vi "uarttest.vi"() -> ()   [LabVIEW 2019]
uses:
  <vilib>/myRIO/Instrument Drivers/Onboard IO/UART/typedef/VISA Configuration.ctl
  KNRm_ReMi_OS6.lvlibp/KNRm_ReMi_Toolkit/IO/LowLevel/IO_Channel_DIO.ctl
  KNRm_ReMi_OS6.lvlibp/KNRm_ReMi_Toolkit/Control/MotorNumberSelect.ctl
  <vilib>/Instr/_visa.llb/VISA Configure Serial Port (Instr).vi
  <vilib>/myRIO/Express VI/Onboard IO/UART/UART Express VI.xnode
  <vilib>/myRIO/Instrument Drivers/Onboard IO/UART/UART.lvlib
  KNRm_ReMi_OS6.lvlibp
  <vilib>/Platform/TimedLoop/XDataNode/XDataNode.xnode
  <vilib>/Platform/TimedLoop/XDataNode/nitl_modes.ctl
  <vilib>/Platform/TimedLoop/XDataNode/XDNodeRunTimeDep.lvlib
  <vilib>/Platform/TimedLoop/XDataNode/wakeup.ctl
  <vilib>/Platform/TimedLoop/XDataNode/timing_clust.ctl
  SJCube_Lib/SJCube Folder/SJCube.lvlib
  <vilib>/addons/control/pid/NI_PID_pid.lvlib
  <vilib>/addons/control/pid/pid.llb/PID (DBL).vi
panel:
  out "Array":string[](array[string])
  out "output":dbl format="%.2f"
  out "Numeric Control":i32
  out "x-y":dbl
  in  "Stop Button 3":bool
  out "Position(deg)":dbl(knob) scale=80.0..-80.0
  in  "Reset":bool
  in  "Stop Button 2":bool
  in  "PosPID":T1={"proportional gain (Kc)"=-0.05999999999999999, "integral time (Ti, min)"=0.03, "derivative time (Td, min)"=0.019999999999999997}
  out "Waveform Chart":T2(graph)
  in  "Setpoint(deg)":dbl(knob) scale=80.0..-80.0
  in  "BalancePID":T1={"proportional gain (Kc)"=0.07999999999999999, "integral time (Ti, min)"=0.0, "derivative time (Td, min)"=0.0008}
  in  "Auto\nSetpoint":bool
  in  "x":bool
  in  "W":string[](array[string])
  out "R":string[](array[string])
  out "ENC(Deg)":dbl
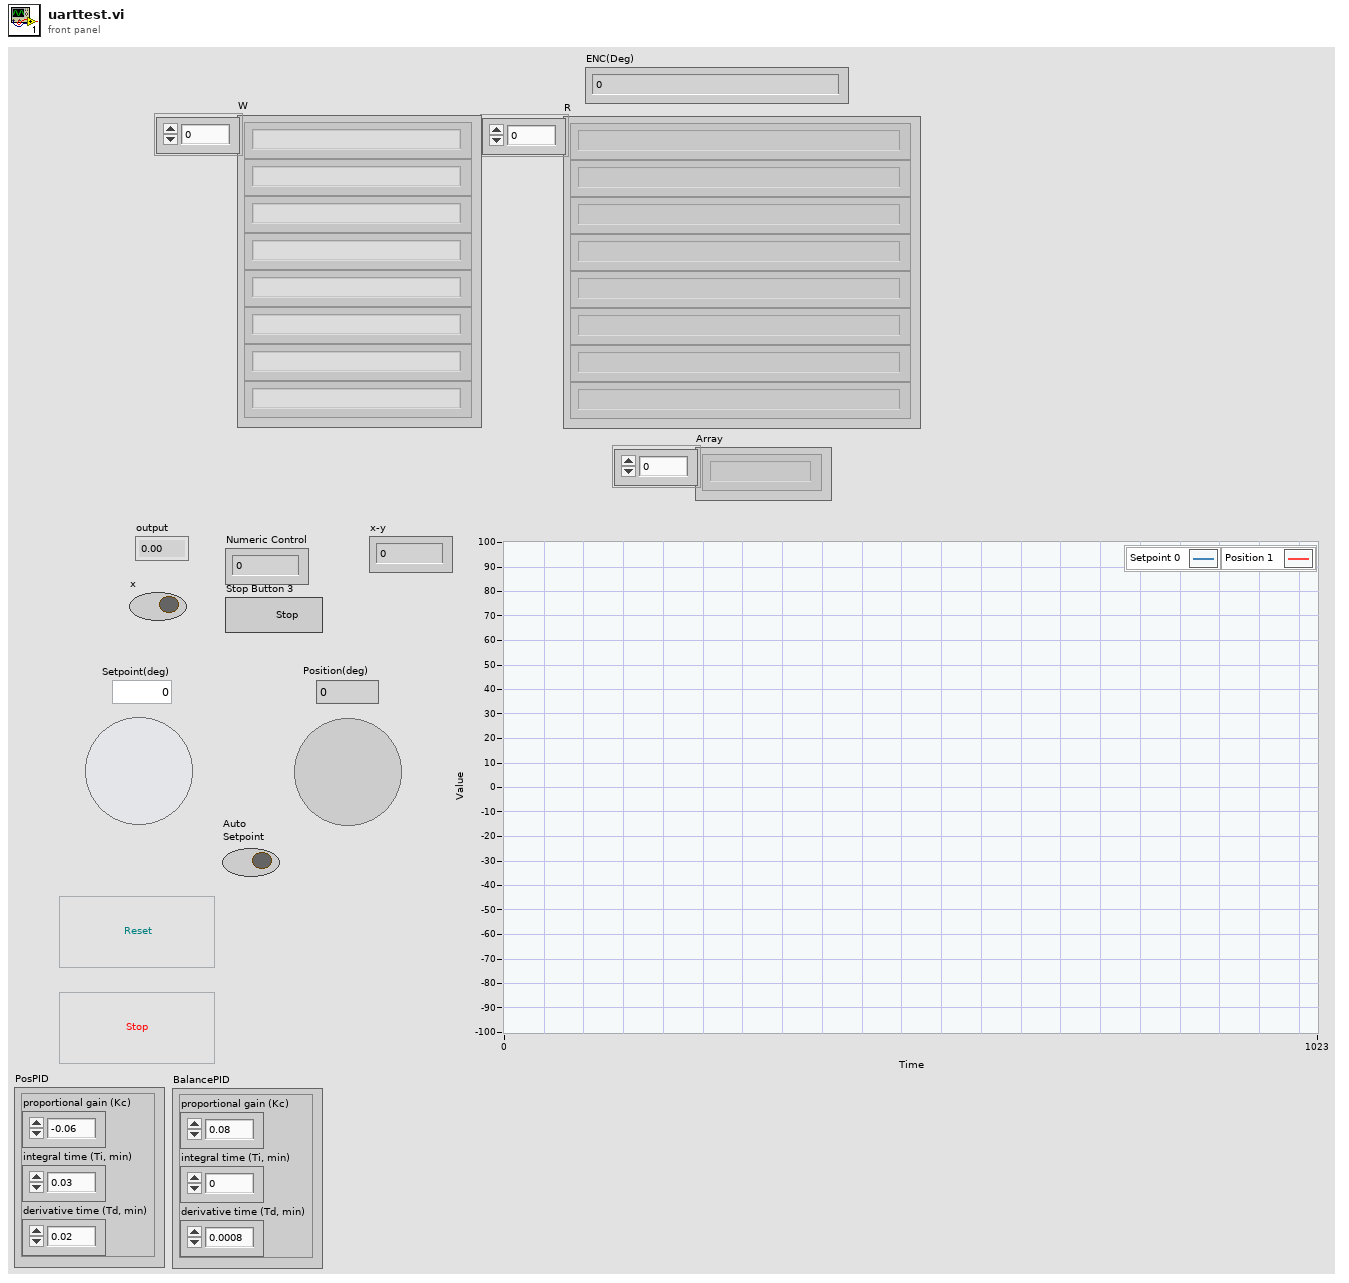
[diagram p1: front panel]
types:
  T1 = cluster{"proportional gain (Kc)":dbl, "integral time (Ti, min)":dbl, "derivative time (Td, min)":dbl}
  T2 = cluster{"Setpoint(deg)":dbl, "PresentPOS(deg)":dbl}
  T3 = typedef "UART.lvlib/VISA Configuration.ctl" = cluster{"baud rate (9600)":u32, "data bits (8)":u16, "parity (0:none)":enum16{"None", "Odd", "Even", "Mark", "Space"}, "stop bits (10: 1 bit)":u16, "flow control (0:none)":u16, "termination char\n(0xA = '\\n' = LF) ":u8, "Enable Termination\nChar (T)":bool, "timeout (10sec)":u32}
  T4 = typedef "KNRm_ReMi_OS6.lvlibp/MotorNumberSelect.ctl" = enum16{"DS1", "DS2", "DS3", "DS4"}
  T5 = typedef "KNRm_ReMi_OS6.lvlibp/IO_Channel_DIO.ctl" = enum16{"B/DIO1 (M1)", "A/DIO8 (M2)", "B/DIO7 (M3)", "A/DIO3 (M4)", "A/DIO14 (RC1_0)", "A/DIO15 (RC1_1)", "A/DIO7(S1)", "A/DIO2(S2)", "A/DIO6(S3)", "A/DIO3(S4)", "A/DIO5(S5)", "A/DIO4(S6)"}
  T6 = typedef "XDNodeRunTimeDep.lvlib/timing_clust.ctl" = cluster{"Expected End [f-1]":u64, "Actual End [f-1]":u64, "Finished Late? [f-1]":bool, "Expected End [i-1]":u64, "Actual End [i-1]":u64, "Finished Late? [i-1]":bool, "Expected Start [i]":u64, "Actual Start [i]":u64, "Expected Start [f]":u64, "Actual Start [f]":u64, "Source Name":string, "Structure Name":string, "Period":i64, "Deadline":i64, "Offset":i64, "Start":i64, "Priority":i32, "Timeout":i32, "Mode":T7, "Wakeup Reason":T8, "Error":errorcluster, "Source Type":string, "Secondary Source Type":string, "Global End Time":u64, "Global Start Time":u64, "Frame Duration":u64, "Iteration Duration":u64, "Assigned CPU":i32, "I/O Scan Engine Mode":u32}
  T7 = typedef "XDNodeRunTimeDep.lvlib/nitl_modes.ctl" = enum32{"No Change", "Process missed periods, maintain original phase", "Discard missed periods, maintain original phase", "Process missed periods, ignore original phase", "Discard missed periods, ignore original phase"}
  T8 = typedef "XDNodeRunTimeDep.lvlib/wakeup.ctl" = enum32{"Normal", "Aborted", "Asynchronous wakeup", "Timing source error", "Timed loop error", "Timeout"}
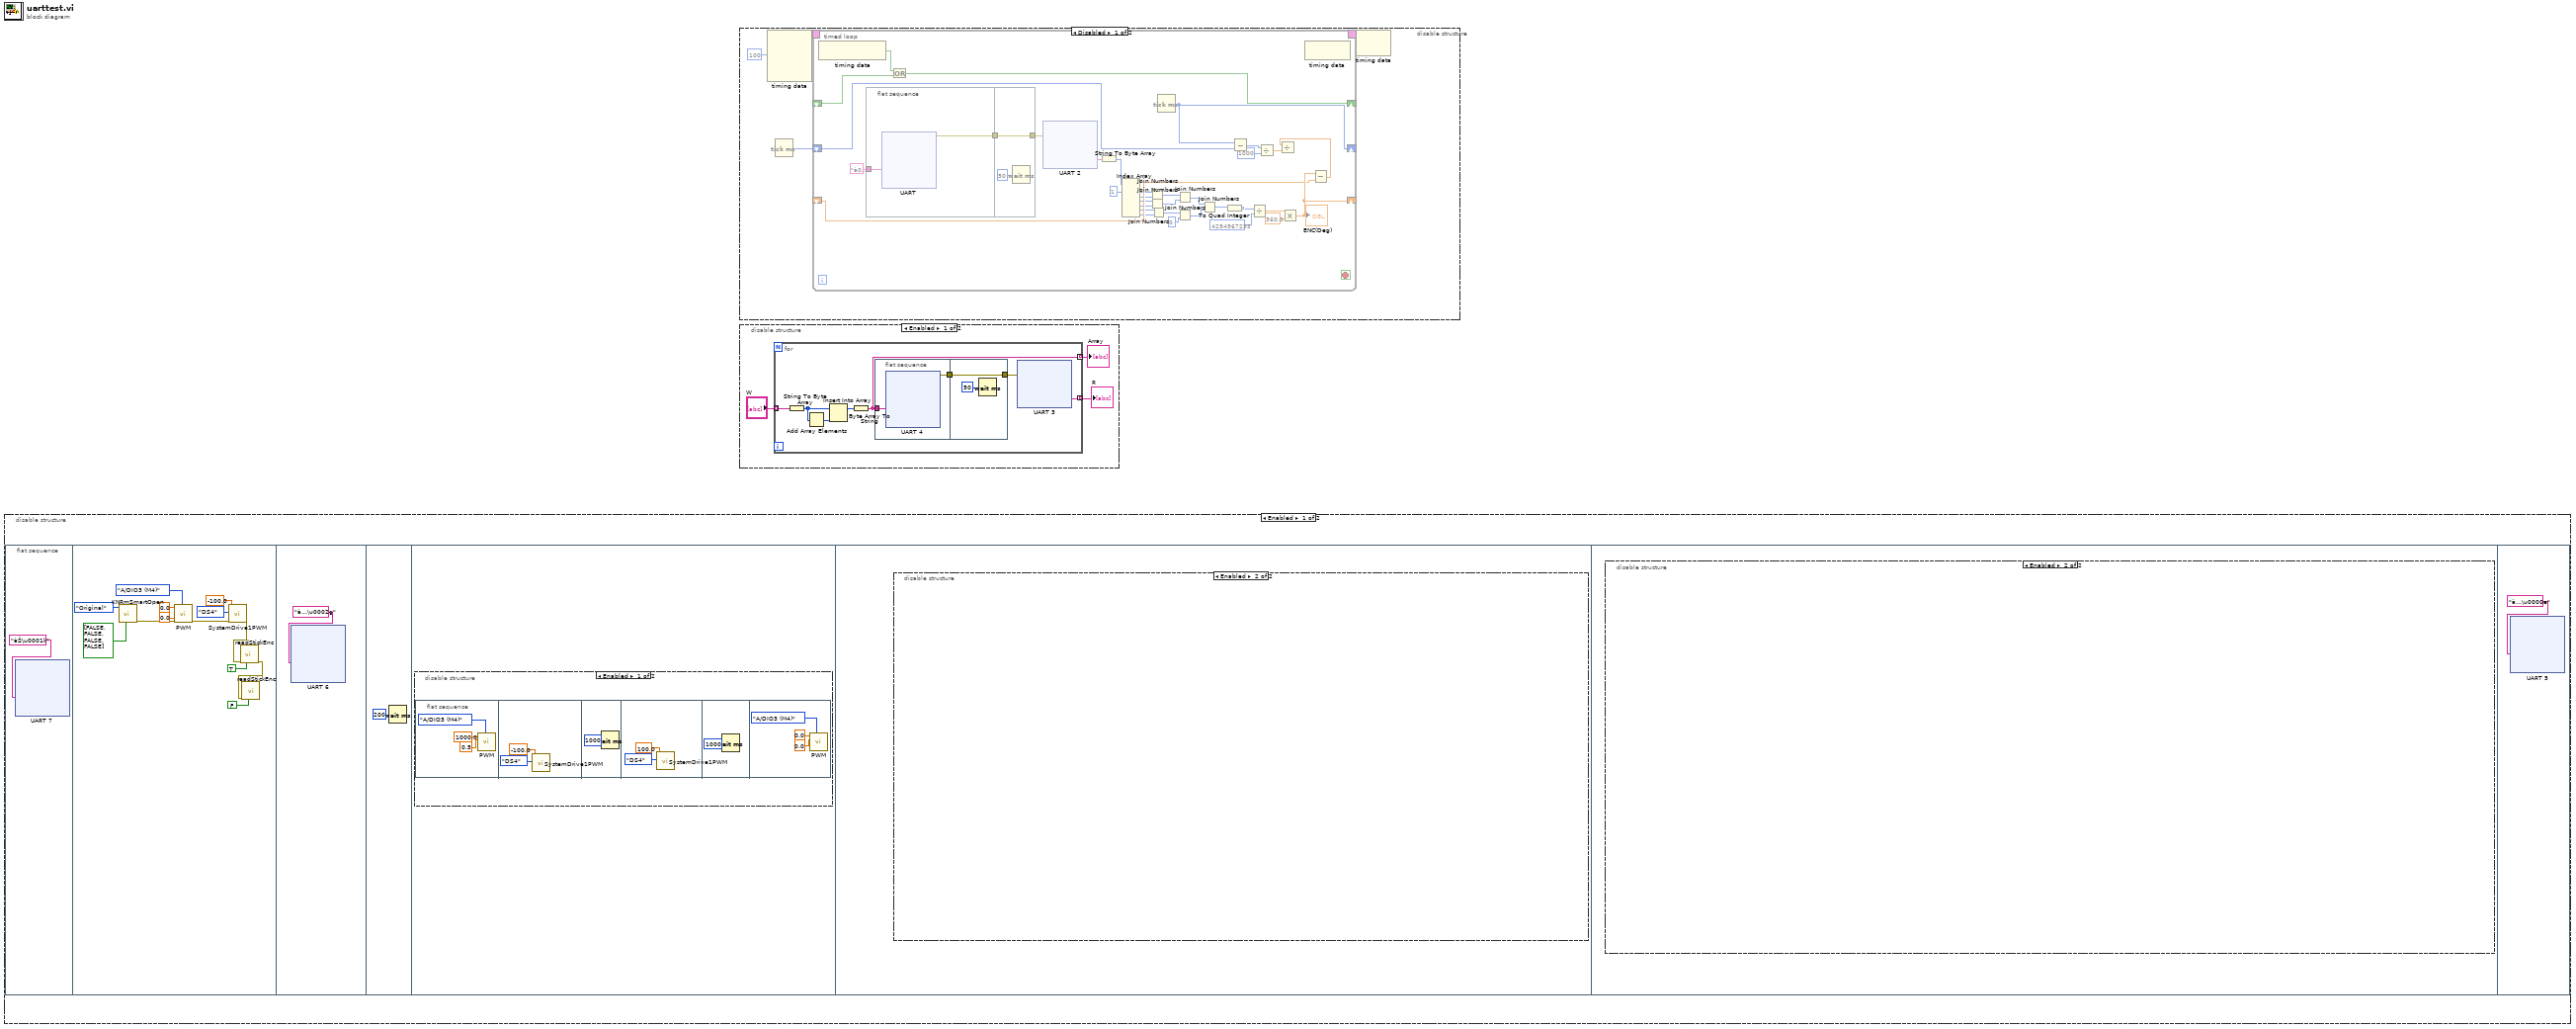
[diagram p0: block diagram]
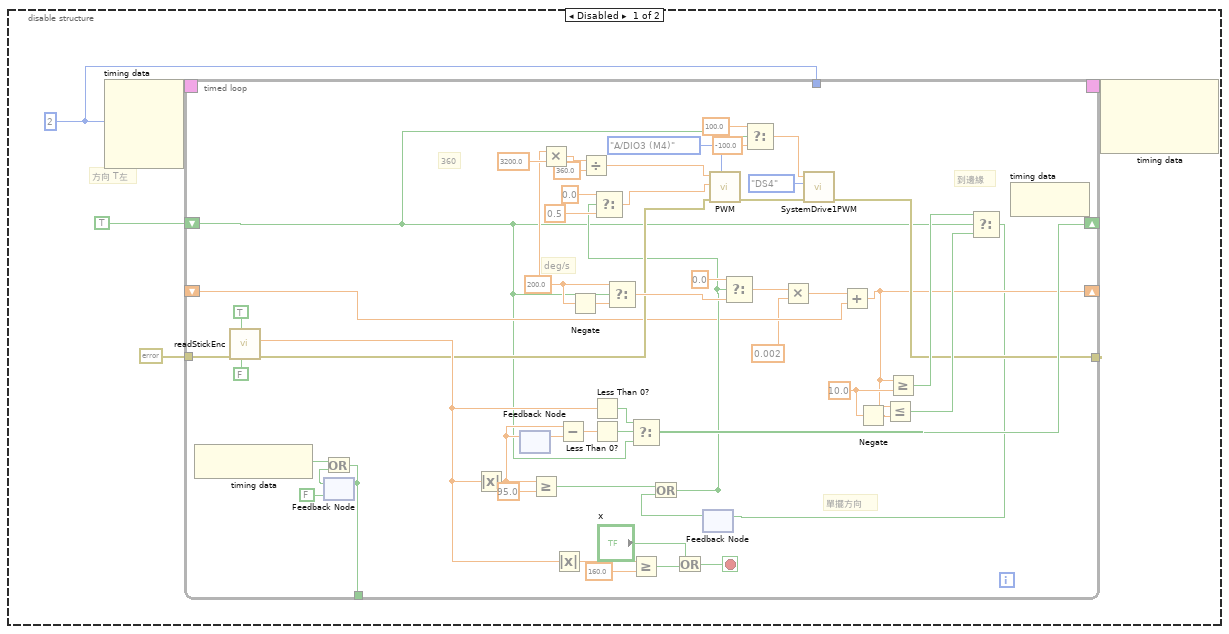
[diagram p3: hidden frame]
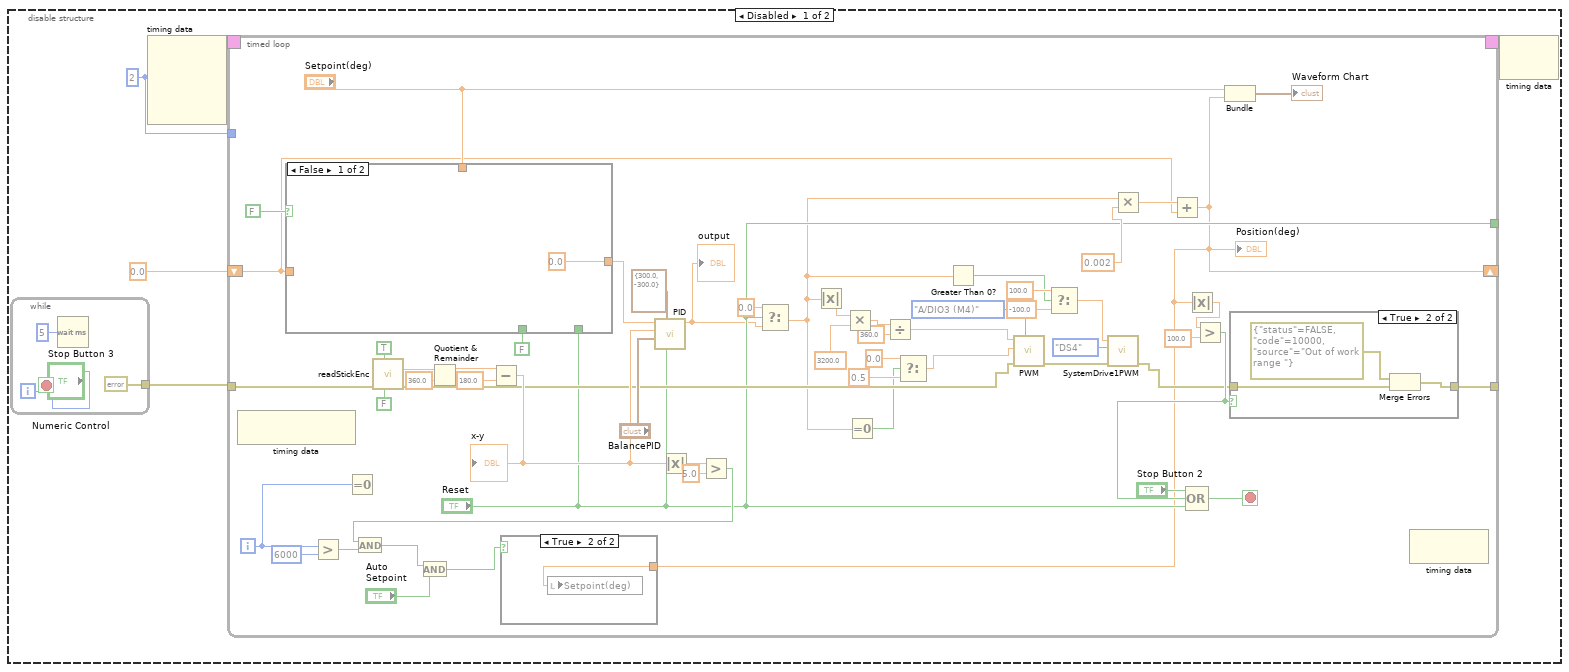
[diagram p4: hidden frame]
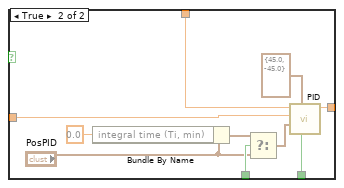
[diagram p6: hidden frame]
diagram:
  n1 = disable-structure shown="Enabled" {
    frame Enabled {
      n2 = flat-sequence {
        frame #0 {
          n3 = xnode "UART 7"("Characters to Write"="àŠ\u0001k" ("string")) -> ()  [unwired: 1 in, 2 out]
        }
        frame #1 {
          n4 = call "KNRmSmartOpen.vi"("SpeedMode"=bool[] [FALSE, FALSE, FALSE, FALSE], "INI FPGA MODE"=enum16{"Original", "M4EXTIOB"}."Original") -> ("error out"=w24:errorcluster)  [unwired: 6 in, 3 out]
          n5 = call "PWM.vi"("IO_Chanel"=IO_Channel_DIO."A/DIO3 (M4)", "error in"=w24, "DutyCycle"=0.0, "Frequency(Hz)"=0.0) -> ("error out"=w23:errorcluster)  [unwired: 7 in]
          n6 = call "SystemDrive1PWM.vi"("error in"=w23, "MotorNumberSelect"=MotorNumberSelect."DS4", "MotorSpeed(PWM%)"=-100.0) -> ("error out"=w29:errorcluster)  [unwired: 7 in, 1 out]
          n7 = call "readStickEnc.vi"("Reset Counter"=TRUE, "error in (no error)"=w29) -> ("error out"=w30:errorcluster)  [unwired: 8 in, 1 out]
          n8 = call "readStickEnc.vi"("Reset Counter"=FALSE, "error in (no error)"=w30) -> ()  [unwired: 8 in, 2 out]
        }
        frame #2 {
          n9 = xnode "UART 6"("Characters to Write"="à…\u0002g" ("string")) -> ()  [unwired: 1 in, 2 out]
        }
        frame #3 {
          n10 = Wait (ms)(milliseconds to wait=u32 200) -> ()  [unwired: 1 out]
        }
        frame #4 {
          n11 = disable-structure shown="Enabled" {
            frame Enabled {
              n12 = flat-sequence {
                frame #0 {
                  n13 = call "PWM.vi"("IO_Chanel"=IO_Channel_DIO."A/DIO3 (M4)", "DutyCycle"=0.5, "Frequency(Hz)"=1000.0) -> ()  [unwired: 8 in, 1 out]
                }
                frame #1 {
                  n14 = call "SystemDrive1PWM.vi"("MotorNumberSelect"=MotorNumberSelect."DS4", "MotorSpeed(PWM%)"=-100.0) -> ()  [unwired: 8 in, 2 out]
                }
                frame #2 {
                  n15 = Wait (ms)(milliseconds to wait=u32 1000) -> ()  [unwired: 1 out]
                }
                frame #3 {
                  n16 = call "SystemDrive1PWM.vi"("MotorNumberSelect"=MotorNumberSelect."DS4", "MotorSpeed(PWM%)"=100.0) -> ()  [unwired: 8 in, 2 out]
                }
                frame #4 {
                  n17 = Wait (ms)(milliseconds to wait=u32 1000) -> ()  [unwired: 1 out]
                }
                frame #5 {
                  n18 = call "PWM.vi"("IO_Chanel"=IO_Channel_DIO."A/DIO3 (M4)", "DutyCycle"=0.0, "Frequency(Hz)"=0.0) -> ()  [unwired: 8 in, 1 out]
                }
              }
            }
            frame Disabled {
            }
          }
        }
        frame #5 {
          n19 = disable-structure shown="Enabled" {
            frame Disabled {
              w61 = i64 2 ("Period")
              # "方向 T左"
              n20 = node-c288(w61) -> (w66:T6)  [unwired: 3 in]
              n21 = timed-loop {
                timing: w66 -> [_]
                timing-out: [_] -> w65
                tunnel: errorcluster {"status"=FALSE, "code"=0, "source"=""} ("error in (no error)") -> [w113]
                tunnel: [w86] -> _
                tunnel: w61 -> [_]
                shift-right: [w100] -> _
                shift-left: TRUE -> [w69]
                tunnel: [w96] -> w64
                shift-right: [w72] -> _
                shift-left: _ -> [w74]
                stop <- w117 stop-if-true
                w95 = 10.0 ("UpLimit")
                w78 = 200.0
                # "360"
                # "deg/s"
                # "單擺方向"
                # "到邊緣"
                n22 = node-c288() -> (w99:bool)  [unwired: 1 in]
                n23 = call "readStickEnc.vi"("Reset Counter"=FALSE, "Reverse ENC?"=TRUE, "error in (no error)"=w113) -> ("error out"=w87:errorcluster, "StickEncoder (deg)"=w93:dbl)  [unwired: 7 in]
                n24 = feedback #1(FALSE) -> (w98:bool)
                n25 = Or(x=w99, y=w98) -> (x .or. y?=w96:bool)
                n26 = feedback-in #1(w96) -> ()
                n27 = Absolute Value(x=w93) -> (abs(x)=w104:dbl)
                n28 = feedback-in #2(w104) -> ()
                n29 = feedback #2() -> (w108:dbl)  [unwired: 1 in]
                n30 = Greater Or Equal?(x=w104, y=95.0) -> (x >= y?=w106:bool)
                n31 = Multiply(x=w78, y=3200.0) -> (x*y=w82:dbl)
                n32 = Absolute Value(x=w93) -> (abs(x)=w119:dbl)
                n33 = Subtract(x=w104, y=w108) -> (x-y=w107:dbl)
                n34 = Negate(x=w78) -> (-x=w110:dbl)
                n35 = Divide(x=w82, y=360.0) -> (x/y=w79:dbl)
                n36 = Less Than 0?(x=w93) -> (x < 0?=w102:bool)
                n37 = Less Than 0?(x=w107) -> (x < 0?=w103:bool)
                n38 = Select(t=w78, s=w69, f=w110) -> (s? t:f=w91:dbl)
                n39 = Select(t=w102, s=w103, f=w69) -> (s? t:f=w100:bool)
                n40 = Greater Or Equal?(x=w119, y=160.0) -> (x >= y?=w101:bool)
                n41 = Or(x="x", y=w101) -> (x .or. y?=w117:bool)
                n42 = feedback #3() -> (w105:bool)  [unwired: 1 in]
                n43 = Or(x=w106, y=w105) -> (x .or. y?=w77:bool)
                n44 = Select(t=0.0, s=w77, f=0.5 ("DutyCycle")) -> (s? t:f=w84:dbl)
                n45 = call "PWM.vi"("IO_Chanel"=IO_Channel_DIO."A/DIO3 (M4)", "error in"=w87, "DutyCycle"=w84, "Frequency(Hz)"=w79) -> ("error out"=w90:errorcluster)  [unwired: 7 in]
                n46 = Select(t=0.0, s=w77, f=w91) -> (s? t:f=w76:dbl)
                n47 = Select(t=100.0, s=w69, f=-100.0) -> (s? t:f=w70:dbl)
                n48 = Multiply(x=w76, y=0.002) -> (x*y=w75:dbl)
                n49 = call "SystemDrive1PWM.vi"("error in"=w90, "MotorNumberSelect"=MotorNumberSelect."DS4", "MotorSpeed(PWM%)"=w70) -> ("error out"=w86:errorcluster)  [unwired: 7 in, 1 out]
                n50 = Add(x=w75, y=w74) -> (x+y=w72:dbl)
                n51 = Negate(x=w95) -> (-x=w94:dbl)
                n52 = Less Or Equal?(x=w72, y=w94) -> (x <= y?=w115:bool)
                n53 = Greater Or Equal?(x=w72, y=w95) -> (x >= y?=w116:bool)
                n54 = Select(t=w116, s=w69, f=w115) -> (s? t:f=w71:bool)
                n55 = feedback-in #3(w71) -> ()
                n56 = node-c288() -> ()  [unwired: 1 in, 1 out]
              }
              n57 = node-c288(w65) -> ()  [unwired: 3 out]
            }
            frame Enabled {
            }
          }
        }
        frame #6 {
          n58 = disable-structure shown="Enabled" {
            frame Disabled {
              w129 = i64 2 ("Period")
              n59 = while {
                tunnel: [errorcluster {"status"=FALSE, "code"=0, "source"=""} ("error out")] -> w127
                i -> [w133]
                stop <- "Stop Button 3" stop-if-true
                n60 = Wait (ms)(milliseconds to wait=u32 5) -> ()  [unwired: 1 out]
                "Numeric Control" <- w133
              }
              n61 = node-c288(w129) -> (w131:T6)  [unwired: 3 in]
              n62 = timed-loop "Timed Loop" {
                timing: w131 -> [_]
                timing-out: [_] -> w130
                shift-right: [w140] -> _
                shift-left: 0.0 -> [w162]
                tunnel: w127 -> [w182]
                tunnel: ["Reset"] -> _
                tunnel: [w180] -> _
                tunnel: w129 -> [_]
                i -> [w166]
                stop <- w186 stop-if-true
                n63 = node-c288() -> ()  [unwired: 1 in, 1 out]
                n64 = case shown="False" FALSE ("StickPosControl") {
                  tunnel: [0.0 ("output") w202] -> w173
                  tunnel: w162 -> [_ w201]
                  tunnel: "Reset" -> [_ w200]
                  tunnel: "Setpoint(deg)" -> [_ w199]
                  tunnel: FALSE -> [_ w198]
                  frame False {
                  }
                  frame True {
                    n65 = Bundle By Name(cluster="PosPID", "integral time (Ti, min)"=0.0) -> (w195:T1)
                    n66 = Select(t=w195, s=w198, f="PosPID") -> (s? t:f=w197:T1)
                    n67 = call-poly <vilib>:"PID.vi"("reinitialize? (F)"=w200, "output range"=cluster{"output high":dbl, "output low":dbl} {"output high"=45.0, "output low"=-45.0}, "PID gains"=w197, "process variable"=w201, "setpoint"=w199) -> ("output"=w202:dbl)  [unwired: 5 in, 1 out]
                  }
                }
                n68 = Greater?(x=w166, y=6000) -> (0:w174:bool)
                n69 = Equal To 0?(x=w166) -> ()  [unwired: 1 out]
                n70 = call "readStickEnc.vi"("Reset Counter"=FALSE, "Reverse ENC?"=TRUE, "error in (no error)"=w182) -> ("error out"=w144:errorcluster, "StickEncoder (deg)"=w184:dbl)  [unwired: 7 in]
                n71 = Quotient & Remainder(x=w184, y=360.0) -> (x-y*floor(x/y)=w187:dbl)  [unwired: 1 out]
                n72 = Subtract(x=w187, y=180.0) -> (x-y=w170:dbl)
                "x-y" <- w170
                n73 = call-poly <vilib>:"PID.vi"("reinitialize? (F)"="Reset", "output range"=cluster{"output high":dbl, "output low":dbl} {"output high"=300.0, "output low"=-300.0}, "PID gains"="BalancePID", "process variable"=w170, "setpoint"=w173) -> ("output"=w136:dbl)  [unwired: 5 in, 1 out]
                "output" <- w136
                n74 = Absolute Value(x=w170) -> (abs(x)=w172:dbl)
                n75 = Greater?(x=w172, y=5.0) -> (0:w165:bool)
                n76 = And(x=w165, y=w174) -> (x .and. y?=w169:bool)
                n77 = And(x=w169, y="Auto\nSetpoint") -> (x .and. y?=w167:bool)
                n78 = Select(t=0.0, s="Reset", f=w136) -> (s? t:f=w138:dbl)
                n79 = Absolute Value(x=w138) -> (abs(x)=w137:dbl)
                n80 = Multiply(x=w137, y=3200.0) -> (x*y=w151:dbl)
                n81 = Equal To 0?(x=w138) -> (x = 0?=w139:bool)
                n82 = Divide(x=w151, y=360.0) -> (x/y=w148:dbl)
                n83 = Select(t=0.0, s=w139, f=0.5 ("DutyCycle")) -> (s? t:f=w153:dbl)
                n84 = Greater Than 0?(x=w138) -> (x > 0?=w142:bool)
                n85 = call "PWM.vi"("IO_Chanel"=IO_Channel_DIO."A/DIO3 (M4)", "error in"=w144, "DutyCycle"=w153, "Frequency(Hz)"=w148) -> ("error out"=w157:errorcluster)  [unwired: 7 in]
                n86 = Select(t=100.0, s=w142, f=-100.0) -> (s? t:f=w147:dbl)
                n87 = call "SystemDrive1PWM.vi"("error in"=w157, "MotorNumberSelect"=MotorNumberSelect."DS4", "MotorSpeed(PWM%)"=w147) -> ("error out"=w143:errorcluster)  [unwired: 7 in, 1 out]
                n88 = Multiply(x=w138, y=0.002) -> (x*y=w163:dbl)
                n89 = Add(x=w163, y=w162) -> (x+y=w140:dbl)
                "Position(deg)" <- w140
                n90 = case shown="True" w167 {
                  tunnel: w140 -> [_ w192]
                  frame False {
                  }
                  frame True {
                    n91 = local write "Setpoint(deg)"(w192) -> ()
                  }
                }
                n92 = Absolute Value(x=w140) -> (abs(x)=w160:dbl)
                n93 = Greater?(x=w160, y=100.0 ("WorkRange")) -> (0:w158:bool)
                n94 = Compound Arithmetic op=OR("Stop Button 2", w158, "Reset") -> (w186:bool)
                n95 = Bundle("Setpoint(deg)"="Setpoint(deg)", w140) -> (→"Waveform Chart":cluster{"Setpoint(deg)":dbl, dbl})  [unwired: 1 in]
                n96 = case shown="True" w158 {
                  tunnel: w143 -> [w204 w207]
                  tunnel: [w204 w205] -> w180
                  frame False {
                  }
                  frame True {
                    n97 = Merge Errors(errorcluster {"status"=FALSE, "code"=10000, "source"="Out of work range "} ("error in (no error)"), w207) -> (w205:errorcluster)
                  }
                }
                n98 = node-c288() -> ()  [unwired: 1 in, 1 out]
              }
              n99 = node-c288(w130) -> ()  [unwired: 1 out]
            }
            frame Enabled {
            }
          }
        }
        frame #7 {
          n100 = xnode "UART 5"("Characters to Write"="à…\u0000e" ("string")) -> ()  [unwired: 1 in, 2 out]
        }
      }
    }
    frame Disabled {
    }
  }
  n101 = disable-structure shown="Disabled" {
    frame Disabled {
      n102 = node-c288(i64 100 ("Period")) -> (w234:T6)  [unwired: 3 in]
      n103 = Tick Count (ms)() -> (millisecond timer value=w232:u32)
      n104 = timed-loop {
        shift-right: [w267] -> _
        shift-left: w232 -> [w268]
        shift-right: [w266] -> _
        shift-left: _ -> [w265]
        timing: w234 -> [_]
        timing-out: [_] -> w233
        shift-right: [w236] -> _
        shift-left: _ -> [w235]
        stop <- _ stop-if-true
        n105 = node-c288() -> (w237:bool)  [unwired: 1 in]
        n106 = flat-sequence {
          tunnel: "à0\u0010" ("string") -> [w270]
          tunnel: [w269] -> w264
          tunnel: [w288] -> w263
          tunnel: w264 -> [w288]
          frame #0 {
            n107 = xnode "UART"("Characters to Write"=w270) -> ("error out"=w269:errorcluster)  [unwired: 1 in, 1 out]
          }
          frame #1 {
            n108 = Wait (ms)(milliseconds to wait=u32 50) -> ()  [unwired: 1 out]
          }
        }
        n109 = Or(x=w237, y=w235) -> (x .or. y?=w236:bool)
        n110 = xnode "UART 2"("error in (no error)"=w263) -> ("Characters Read"=w262:string)  [unwired: 1 out]
        n111 = String To Byte Array(string=w262) -> (unsigned byte array=w261:u8[])
        n112 = Index Array(array=w261, index #1=1 ("index")) -> (element #1=w257:u8, element #2=w256:u8, element #3=w255:u8, element #4=w254:u8, element #5=w253:u8, element #6=w252:u8)  [unwired: 5 in]
        n113 = Join Numbers(hi=w257, lo=w256) -> ((hi.lo)=w251:u16)
        n114 = Join Numbers(hi=w255, lo=w254) -> ((hi.lo)=w250:u16)
        n115 = Join Numbers(hi=w253, lo=w252) -> ((hi.lo)=w249:u16)
        n116 = Tick Count (ms)() -> (millisecond timer value=w267:u32)
        n117 = Join Numbers(hi=w251, lo=w250) -> ((hi.lo)=w259:u32)
        n118 = Join Numbers(hi=w249, lo=u16 0) -> ((hi.lo)=w258:u32)
        n119 = Join Numbers(hi=w259, lo=w258) -> ((hi.lo)=w247:u64)
        n120 = To Quad Integer(1:w247) -> (0:w243:i64)
        n121 = Subtract(x=w267, y=w268) -> (x-y=w241:u32)
        n122 = Divide(x=w243, y=i64 4294967295) -> (x/y=w245:dbl)
        n123 = Divide(x=w241, y=u32 1000) -> (x/y=w239:dbl)
        n124 = Multiply(x=w245, y=360.0) -> (x*y=w266:dbl)
        "ENC(Deg)" <- w266
        n125 = node-c288() -> ()  [unwired: 1 in, 1 out]
        n126 = Subtract(x=w266, y=w265) -> (x-y=w238:dbl)
        n127 = Divide(x=w238, y=w239) -> ()  [unwired: 1 out]
      }
      n128 = node-c288(w233) -> ()  [unwired: 1 out]
    }
    frame Enabled {
    }
  }
  n129 = disable-structure shown="Enabled" {
    frame Enabled {
      n130 = for {
        tunnel: [w319] -> w314 mode=indexing
        tunnel: "W" -> [w317] mode=indexing
        tunnel: [w316] -> w313 mode=indexing
        n131 = String To Byte Array(string=w317) -> (unsigned byte array=w318:u8[])
        n132 = Add Array Elements(numeric array=w318) -> (sum=w322:u8)
        n133 = Insert Into Array(array=w318, new element=w322) -> (w321:u8[])  [unwired: 1 in]
        n134 = Byte Array To String(unsigned byte array=w321) -> (string=w316:string)
        n135 = flat-sequence {
          tunnel: w316 -> [w325]
          tunnel: [w324] -> w323
          tunnel: [w343] -> w320
          tunnel: w323 -> [w343]
          frame #0 {
            n136 = xnode "UART 4"("Characters to Write"=w325) -> ("error out"=w324:errorcluster)  [unwired: 1 in, 1 out]
          }
          frame #1 {
            n137 = Wait (ms)(milliseconds to wait=u32 50) -> ()  [unwired: 1 out]
          }
        }
        n138 = xnode "UART 3"("error in (no error)"=w320) -> ("Characters Read"=w319:string)  [unwired: 1 out]
      }
      "R" <- w314
      "Array" <- w313
    }
    frame Disabled {
    }
  }
